vi "LabelWires.vi"(4 "Error In":errorcluster, 7 "DAQ Raw Measurement Array":dbl[](array[numeric])) -> (0 "Error Out":errorcluster, 3 "Named DAQ Cluster":T1)   [LabVIEW 2012]
panel:
  in  "Data Organization Cluster":T1
  # "Label the Wires Coming from the DAQ"
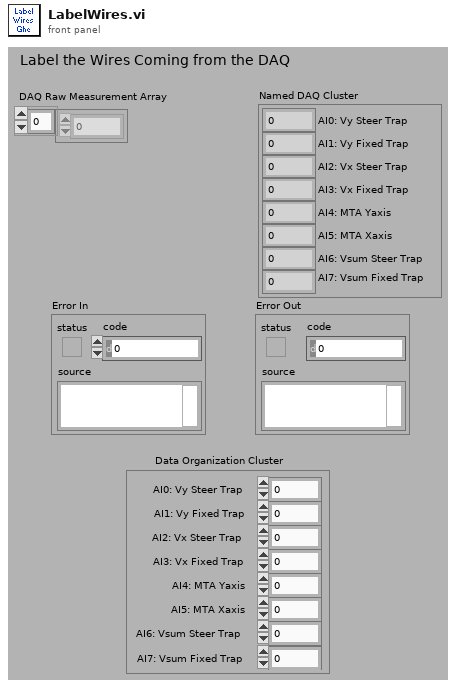
[diagram p1: front panel]
types:
  T1 = cluster{"AI0: Vy Steer Trap":dbl, "AI1: Vy Fixed Trap":dbl, "AI2: Vx Steer Trap":dbl, "AI3: Vx Fixed Trap":dbl, "AI4: MTA Yaxis":dbl, "AI5: MTA Xaxis":dbl, "AI6: Vsum Steer Trap":dbl, "AI7: Vsum Fixed Trap":dbl}
  T2 = cluster{"DAQ Raw Measurement Array[0]":dbl, "DAQ Raw Measurement Array[1]":dbl, "DAQ Raw Measurement Array[2]":dbl, "DAQ Raw Measurement Array[3]":dbl, "DAQ Raw Measurement Array[4]":dbl, "DAQ Raw Measurement Array[5]":dbl, "DAQ Raw Measurement Array[6]":dbl, "DAQ Raw Measurement Array[7]":dbl}
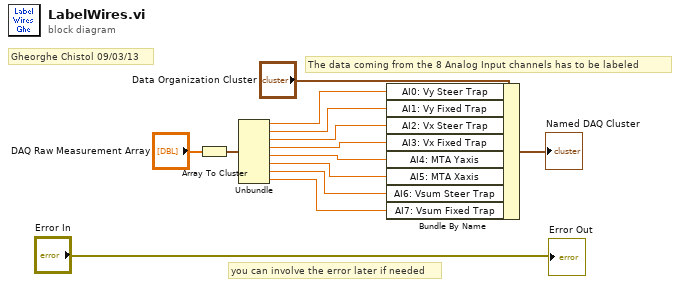
[diagram p0: block diagram]
diagram:
  # "you can involve the error later if needed"
  # "Gheorghe Chistol 09/03/13"
  # "The data coming from the 8 Analog Input channels has to be labeled"
  n1 = Array To Cluster(array="DAQ Raw Measurement Array") -> (cluster=w12:T2)
  n2 = Unbundle(w12) -> ("DAQ Raw Measurement Array[0]"=w10:dbl, "DAQ Raw Measurement Array[1]"=w9:dbl, "DAQ Raw Measurement Array[2]"=w8:dbl, "DAQ Raw Measurement Array[3]"=w7:dbl, "DAQ Raw Measurement Array[4]"=w6:dbl, "DAQ Raw Measurement Array[5]"=w5:dbl, "DAQ Raw Measurement Array[6]"=w4:dbl, "DAQ Raw Measurement Array[7]"=w3:dbl)
  n3 = Bundle By Name(cluster="Data Organization Cluster", "AI0: Vy Steer Trap"=w10, "AI1: Vy Fixed Trap"=w9, "AI2: Vx Steer Trap"=w8, "AI3: Vx Fixed Trap"=w7, "AI4: MTA Yaxis"=w6, "AI5: MTA Xaxis"=w5, "AI6: Vsum Steer Trap"=w4, "AI7: Vsum Fixed Trap"=w3) -> (→"Named DAQ Cluster":T1)
  "Error Out" <- "Error In"
